vi "ReadSalicruAPI (SubVI).vi"(8 "error in (no error)":errorcluster, 10 "Python File":path, 11 "session in":refnum<k35>) -> (0 "error out":errorcluster, 1 "Array":i32[](array[numeric]), 2 "Map":map{string, dbl}(c390), 3 "session out":refnum<k35>)   [LabVIEW 2024]
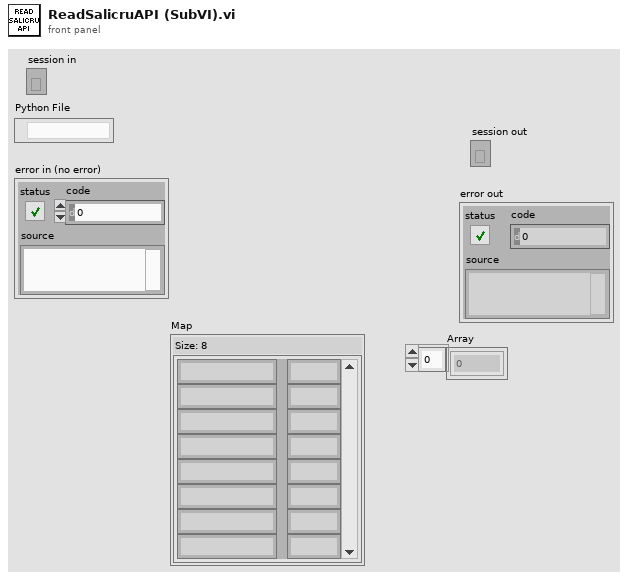
[diagram p1: front panel]
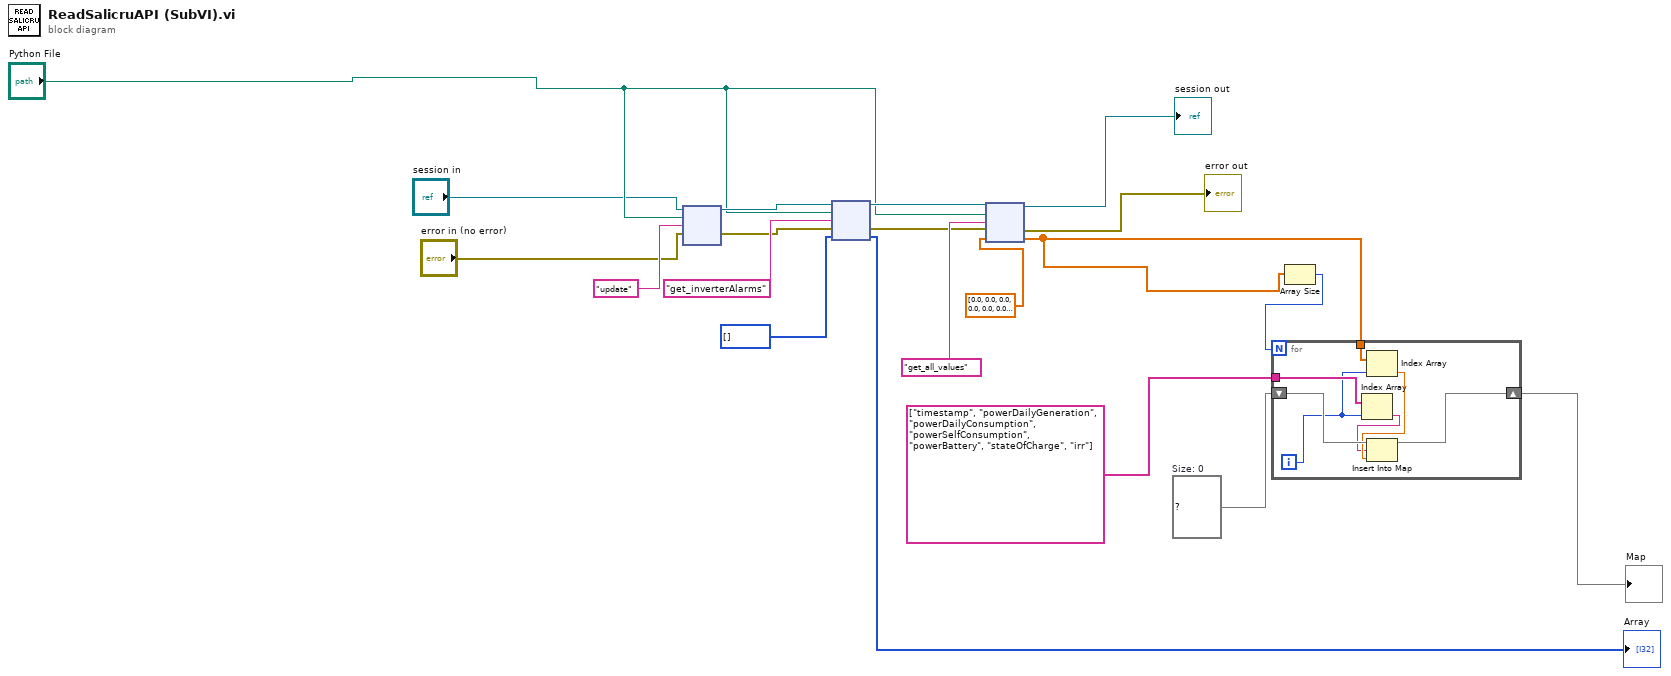
[diagram p0: block diagram]
diagram:
  w17 = map{string, dbl} {}  # Size: 0
  n1 = node("session in", "Python File", "update" ("function name"), "error in (no error)") -> (w7:refnum<k35>, w8:errorcluster)  [unwired: 2 in, 2 out]
  n2 = node(w7, "Python File", "get_inverterAlarms" ("function name"), w8, i32[] []) -> (w10:refnum<k35>, w11:errorcluster, →"Array":i32[])  [unwired: 2 out]
  n3 = node(w10, "Python File", "get_all_values" ("function name"), w11, dbl[] [0.0, 0.0, 0.0, 0.0, 0.0, 0.0, 0.0, 0.0]) -> (→"session out":refnum<k35>, →"error out":errorcluster, w18:dbl[])  [unwired: 2 out]
  n4 = Array Size(array=w18) -> (size(s)=w16:i32)
  n5 = for {
    N: w16 -> [_]
    shift-right: [w27] -> w20
    shift-left: w17 -> [w26]
    tunnel: w18 -> [w25]
    tunnel: string[] ["timestamp", "powerDailyGeneration", "powerDailyConsumption", "powerSelfConsumption", "powerBattery", "stateOfCharge", "irr"] -> [w24]
    i -> [w23]
    n6 = Index Array(array=w24, index=w23) -> (element=w21:string)
    n7 = Index Array(array=w25, index=w23) -> (element=w22:dbl)
    n8 = Insert Into Map(map in=w26, key=w21, value=w22) -> (map out=w27:map{string, dbl})  [unwired: 2 out]
  }
  "Map" <- w20
